vi "Periodic Tasks.vi"(8 "error in":errorcluster) -> ()   [LabVIEW 2013]
doc: "This VI runs in parallel to other tasks. It can contain as many user-defined periodic loops as you need. These can carry out PID or other sorts of timed response."
uses:
  <vilib>/Rock Robotics/SystemInterfaces/Utilities/FPGA_UtilitiesLED Source.ctl
  <vilib>/Rock Robotics/SystemInterfaces/Utilities/FPGA_UtilitiesLED State.ctl
  <vilib>/Rock Robotics/WPI/Relay/WPI_RelayValue.ctl
  <vilib>/Rock Robotics/WPI/Compressor/WPI_CompressorGetSetRefNum.vi
  Robot Global Data.vi
  <vilib>/Rock Robotics/WPI/RobotDrive/WPI_RobotDriveGetSetRefNum.vi
  <vilib>/Rock Robotics/WPI/Joystick/WPI_JoystickGetSetRefNum.vi
panel:
  out "Timings":cluster{"Call Name":string, "Delta (ms)":u32}[](array[cluster])
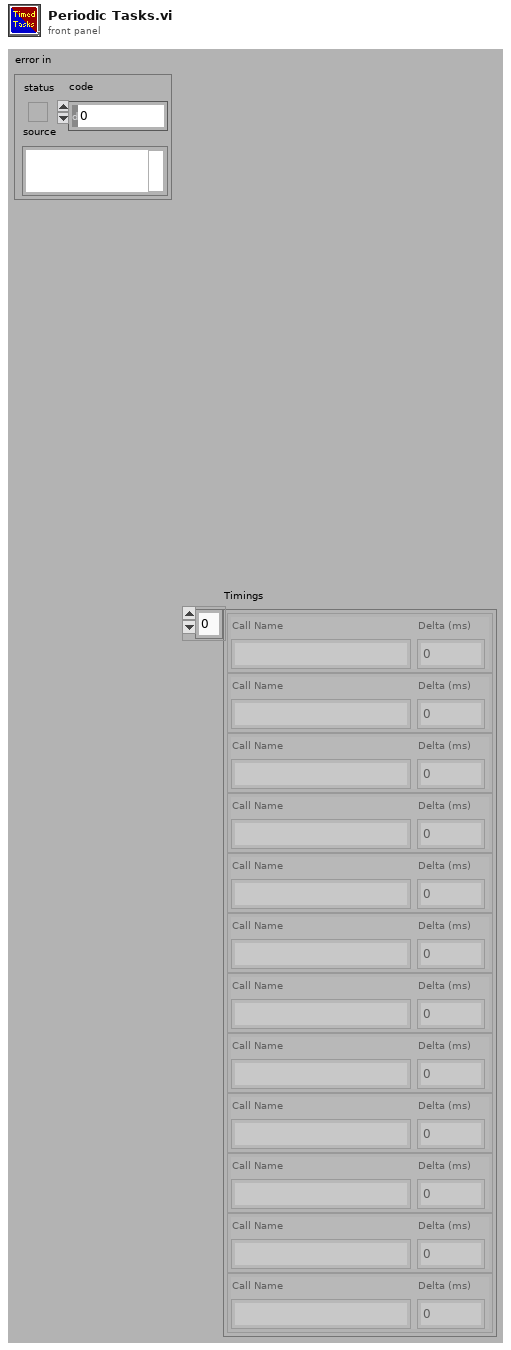
[diagram p1: front panel]
types:
  T1 = typedef "WPI_JoystickDevRef.ctl" = cluster{"Device":T2}
  T2 = typedef "WPI_JoystickDeviceEnum.ctl" = enum16{"USB 1", "USB 2", "USB 3", "USB 4", "Kinect 1", "Kinect 2"}
  T3 = typedef "WPI_RobotDriveDevRef.ctl" = cluster{"DevStatus":errorcluster, "Motors[]":T4[], "Square Inputs":bool, "Max Output":dbl, "Isochronous":bool}
  T4 = typedef "WPI_MotorControlDeviceRef.ctl" = cluster{"DeviceStatus":errorcluster, "Type":enum16{"PWM", "CAN"}, "PWM":cluster{"Digital Module":T5, "PWM Channel":T6, "DeadBand":T7}, "CAN":cluster{"Device Number":u8, "Control Mode":T8, "Semaphore":T9, "Max Vout":dbl}, "Invert":bool, "TransformRef":T10, "InvTransformRef":T10}
  T5 = typedef "FPGA_TypedefDigitalModule.ctl" = enum16{"Digital Module 1", "Digital Module 2"}
  T6 = typedef "FPGA_DIOPWMChannel.ctl" = enum8{"PWM 1", "PWM 2", "PWM 3", "PWM 4", "PWM 5", "PWM 6", "PWM 7", "PWM 8", "PWM 9", "PWM 10", "Invalid"}
  T7 = typedef "WPI_PWMDeadband.ctl" = cluster{"Name":string, "maxPositivePwm":i32, "minPositivePwm":i32, "centerPwm":i32, "maxNegativePwm":i32, "minNegativePwm":i32, "angularRange":u16}
  T8 = typedef "WPI_CANJaguar_ControlMode.ctl" = enum8{"Percent VBus", "Current", "Speed", "Position", "Voltage"}
  T9 = typedef "Semaphore RefNum" = refnum<k1>
  T10 = typedef "WPI_PWMTransform_ConPane.ctl" = refnum<vi>
  T11 = cluster{"JoystickDevRef":T1, "RobotDriveDevRef":T3}
  T12 = typedef "WPI_RelayValue.ctl" = enum16{"Off", "On", "Forward", "Reverse"}
  T13 = typedef "WPI_DriverStationAllianceInfo.ctl" = enum16{"Red", "Blue", "Invalid"}
  T14 = typedef "WPI_RelayDevRef.ctl" = cluster{"DevStatus":errorcluster, "Relay Channel":T15, "Digital Module":T5, "Relay Direction":T16}
  T15 = typedef "FPGA_DIORelayChannel.ctl" = enum8{"Relay 1", "Relay 2", "Relay 3", "Relay 4", "Relay 5", "Relay 6", "Relay 7", "Relay 8", "Invalid"}
  T16 = typedef "WPI_RelayDirection.ctl" = enum16{"Both directions", "Forward only", "Reverse only"}
  T17 = typedef "WPI_CompressorDevRef.ctl" = cluster{"DevStatus":errorcluster, "DigitalInputDevRef":T18, "RelayDevRef":T14}
  T18 = typedef "WPI_DigitalInputDevRef.ctl" = cluster{"DevStatus":errorcluster, "DIO Channel":T19, "Digital Module":T5}
  T19 = typedef "FPGA_DIOChannel.ctl" = enum8{"DIO 1", "DIO 2", "DIO 3", "DIO 4", "DIO 5", "DIO 6", "DIO 7", "DIO 8", "DIO 9", "DIO 10", "DIO 11", "DIO 12", "DIO 13", "DIO 14", "Invalid"}
  T20 = typedef "WPI_JoystickButtonState.ctl" = cluster{"Button 1":bool, "Button 2":bool, "Button 3":bool, "Button 4":bool, "Button 5":bool, "Button 6":bool, "Button 7":bool, "Button 8":bool, "Button 9":bool, "Button 10":bool, "Button 11":bool, "Button 12":bool}
  T21 = cluster{"axis 1 (x)":dbl, "axis 2 (y)":dbl, "axis 3 (throttle)":dbl, "axis 4":dbl, "axis 5":dbl, "axis 6":dbl}
  T22 = typedef "FPGA_UtilitiesLED State.ctl" = enum16{"Off", "On", "Toggle"}
  T23 = typedef "FPGA_UtilitiesLED Source.ctl" = enum16{"User LED", "FPGA LED"}
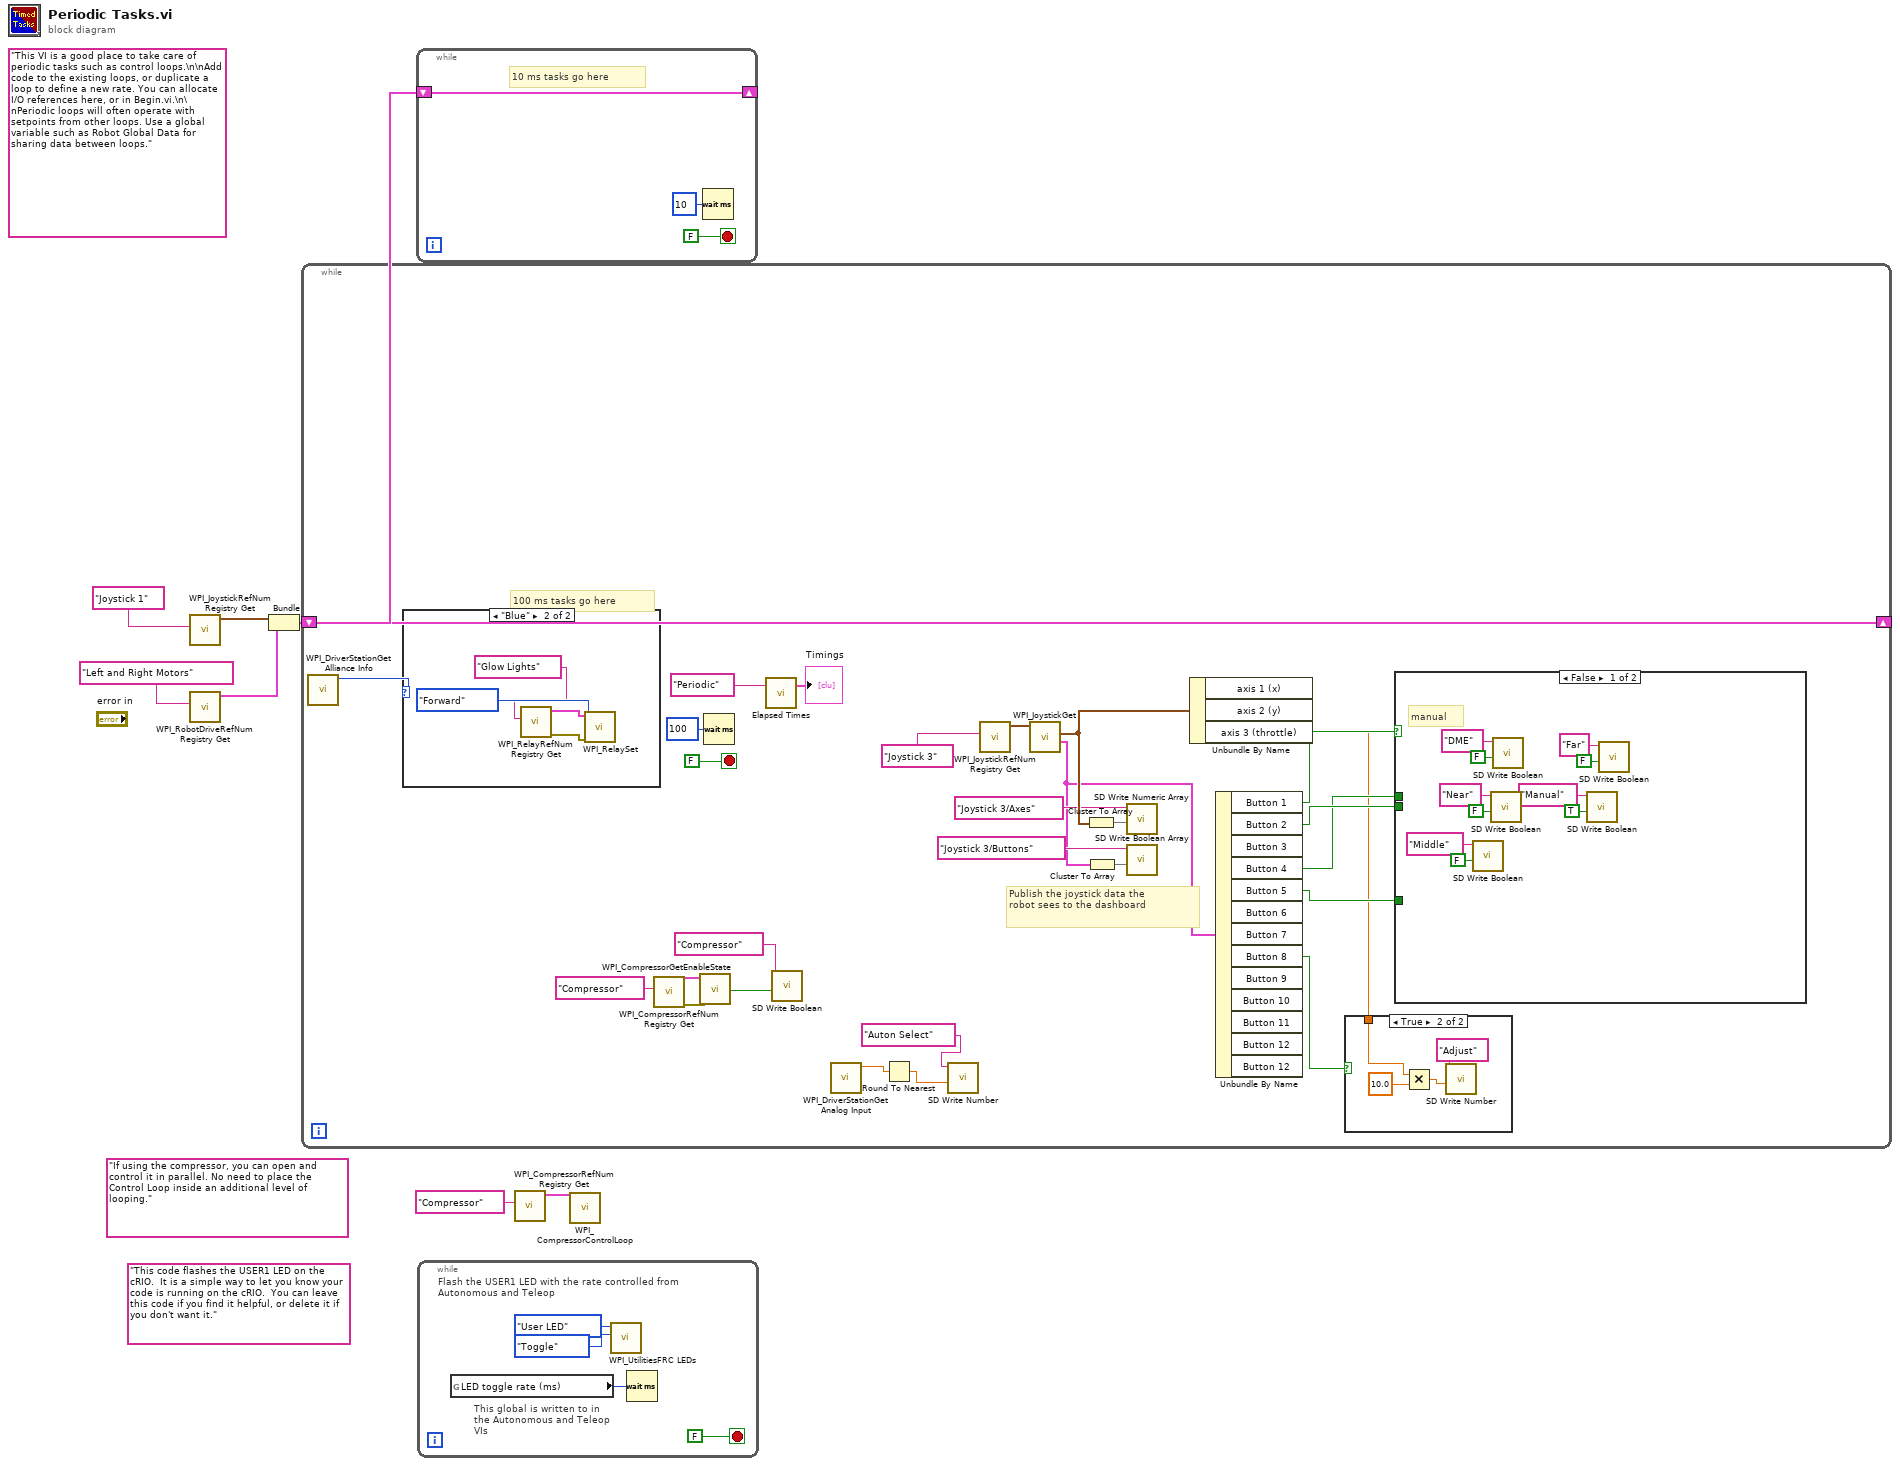
[diagram p0: block diagram]
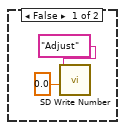
[diagram p2: hidden frame]
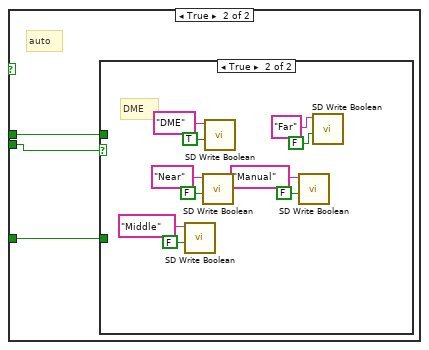
[diagram p3: hidden frame]
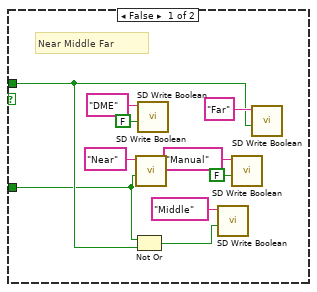
[diagram p4: hidden frame]
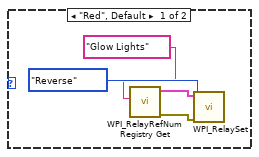
[diagram p5: hidden frame]
diagram:
  (unwired) "If using the compressor, you can open and control it in parallel. No need to place the Control Loop inside an additional level of looping."
  (unwired) "This code flashes the USER1 LED on the cRIO.  It is a simple way to let you know your code is running on the cRIO.  You can leave this code if you find it helpful, or delete it if you don't want it."
  (unwired) "This VI is a good place to take care of periodic tasks such as control loops.\n\nAdd code to the existing loops, or duplicate a loop to define a new rate. You can allocate I/O references here, or in Begin.vi.\n\nPeriodic loops will often operate with setpoints from other loops. Use a global variable such as Robot Global Data for sharing data between loops."
  n1 = call <vilib>:"WPI_JoystickRefNum Registry Get.vi"("refnum name"="Joystick 1") -> ("JoystickDevRef"=w5:T1)  [unwired: 1 in, 9 out]
  n2 = call <vilib>:"WPI_RobotDriveRefNum Registry Get.vi"("refnum name"="Left and Right Motors") -> ("RobotDriveDevRef"=w4:T3)  [unwired: 1 in, 9 out]
  n3 = Bundle("JoystickDevRef"=w5, "RobotDriveDevRef"=w4) -> (w3:T11)  [unwired: 1 out]
  n4 = while {
    shift-right: [w33] -> _
    shift-left: w3 -> [w33]
    stop <- FALSE stop-if-true
    # "Publish the joystick data the\nrobot sees to the dashboard"
    # "100 ms tasks go here"
    n5 = call <vilib>:"WPI_DriverStationGet Alliance Info.vi"() -> ("Alliance"=w32:T13)  [unwired: 10 in, 1 out]
    n6 = case shown="\"Blue\"" w32 {
      frame "Red", Default {
        n7 = call <vilib>:"WPI_RelayRefNum Registry Get.vi"("refnum name"="Glow Lights") -> ("error out"=w77:errorcluster, "RelayDevRef"=w76:T14)  [unwired: 9 in]
        n8 = call <vilib>:"WPI_RelaySet.vi"("error in (no error)"=w77, "RelayValue"=WPI_RelayValue."Reverse", "RelayDevRef"=w76) -> ()  [unwired: 7 in, 2 out]
      }
      frame "Blue" {
        n9 = call <vilib>:"WPI_RelayRefNum Registry Get.vi"("refnum name"="Glow Lights") -> ("error out"=w81:errorcluster, "RelayDevRef"=w80:T14)  [unwired: 9 in]
        n10 = call <vilib>:"WPI_RelaySet.vi"("error in (no error)"=w81, "RelayValue"=WPI_RelayValue."Forward", "RelayDevRef"=w80) -> ()  [unwired: 7 in, 2 out]
      }
    }
    n11 = call <vilib>:"WPI_CompressorRefNum Registry Get.vi"("refnum name"="Compressor") -> ("error out"=w12:errorcluster, "CompressorDevRef"=w11:T17)  [unwired: 9 in]
    n12 = call <vilib>:"WPI_CompressorGetEnableState.vi"("error in (no error)"=w12, "CompressorDevRef"=w11) -> ("Compressor Running"=w9:bool)  [unwired: 6 in, 3 out]
    n13 = Wait (ms)(milliseconds to wait=u32 100) -> ()  [unwired: 1 out]
    n14 = call "Elapsed Times.vi"("Call Name"="Periodic") -> ("Timings"=→"Timings":cluster{"Call Name":string, "Delta (ms)":u32}[])  [unwired: 2 in]
    n15 = call <vilib>:"SD Write Boolean.vi"("Boolean"=w9, "Name"="Compressor") -> ()  [unwired: 8 in, 2 out]
    n16 = call <vilib>:"WPI_DriverStationGet Analog Input.vi"() -> ("Analog 1 (V)"=w16:dbl)  [unwired: 8 in, 3 out]
    n17 = Round To Nearest(number=w16) -> (nearest integer value=w15:dbl)
    n18 = call <vilib>:"SD Write Number.vi"("Numeric"=w15, "Name"="Auton Select") -> ()  [unwired: 8 in, 2 out]
    n19 = call <vilib>:"WPI_JoystickRefNum Registry Get.vi"("refnum name"="Joystick 3") -> ("JoystickDevRef"=w28:T1)  [unwired: 1 in, 9 out]
    n20 = call <vilib>:"WPI_JoystickGet.vi"("JoystickDevRef"=w28) -> ("Buttons"=w22:T20, "Axes"=w25:T21)  [unwired: 1 in, 4 out]
    n21 = Cluster To Array(cluster=w25) -> (array=w24:dbl[])
    n22 = Cluster To Array(cluster=w22) -> (array=w27:bool[])
    n23 = call <vilib>:"SD Write Numeric Array.vi"("Numeric Array"=w24, "Name"="Joystick 3/Axes") -> ()  [unwired: 8 in, 2 out]
    n24 = call <vilib>:"SD Write Boolean Array.vi"("Boolean Array"=w27, "Name"="Joystick 3/Buttons") -> ()  [unwired: 8 in, 2 out]
    n25 = Unbundle By Name(w25) -> ("axis 3 (throttle)"=w13:dbl)  [unwired: 2 out]
    n26 = Unbundle By Name(w22) -> ("Button 1"=w21:bool, "Button 2"=w20:bool, "Button 4"=w18:bool, "Button 5"=w19:bool, "Button 8"=w17:bool)  [unwired: 8 out]
    n27 = case shown="True" w17 {
      tunnel: w13 -> [_ w38]
      frame False {
        n28 = call <vilib>:"SD Write Number.vi"("Numeric"=0.0, "Name"="Adjust") -> ()  [unwired: 8 in, 2 out]
      }
      frame True {
        n29 = Multiply(x=w38, y=10.0) -> (x*y=w41:dbl)
        n30 = call <vilib>:"SD Write Number.vi"("Numeric"=w41, "Name"="Adjust") -> ()  [unwired: 8 in, 2 out]
      }
    }
    n31 = case shown="False" w21 {
      tunnel: w20 -> [_ w54]
      tunnel: w19 -> [_ w53]
      tunnel: w18 -> [_ w52]
      frame False {
        # "manual"
        n32 = call <vilib>:"SD Write Boolean.vi"("Boolean"=FALSE, "Name"="Middle") -> ()  [unwired: 8 in, 2 out]
        n33 = call <vilib>:"SD Write Boolean.vi"("Boolean"=FALSE, "Name"="Near") -> ()  [unwired: 8 in, 2 out]
        n34 = call <vilib>:"SD Write Boolean.vi"("Boolean"=FALSE, "Name"="DME") -> ()  [unwired: 8 in, 2 out]
        n35 = call <vilib>:"SD Write Boolean.vi"("Boolean"=TRUE, "Name"="Manual") -> ()  [unwired: 8 in, 2 out]
        n36 = call <vilib>:"SD Write Boolean.vi"("Boolean"=FALSE, "Name"="Far") -> ()  [unwired: 8 in, 2 out]
      }
      frame True {
        # "auto"
        n37 = case shown="True" w54 {
          tunnel: w53 -> [w56 _]
          tunnel: w52 -> [w57 _]
          frame False {
            # "Near Middle Far"
            n38 = Not Or(1:w57, 2:w56) -> (0:w58:bool)
            n39 = call <vilib>:"SD Write Boolean.vi"("Boolean"=w56, "Name"="Near") -> ()  [unwired: 8 in, 2 out]
            n40 = call <vilib>:"SD Write Boolean.vi"("Boolean"=FALSE, "Name"="DME") -> ()  [unwired: 8 in, 2 out]
            n41 = call <vilib>:"SD Write Boolean.vi"("Boolean"=w58, "Name"="Middle") -> ()  [unwired: 8 in, 2 out]
            n42 = call <vilib>:"SD Write Boolean.vi"("Boolean"=FALSE, "Name"="Manual") -> ()  [unwired: 8 in, 2 out]
            n43 = call <vilib>:"SD Write Boolean.vi"("Boolean"=w57, "Name"="Far") -> ()  [unwired: 8 in, 2 out]
          }
          frame True {
            # "DME"
            n44 = call <vilib>:"SD Write Boolean.vi"("Boolean"=FALSE, "Name"="Middle") -> ()  [unwired: 8 in, 2 out]
            n45 = call <vilib>:"SD Write Boolean.vi"("Boolean"=FALSE, "Name"="Near") -> ()  [unwired: 8 in, 2 out]
            n46 = call <vilib>:"SD Write Boolean.vi"("Boolean"=TRUE, "Name"="DME") -> ()  [unwired: 8 in, 2 out]
            n47 = call <vilib>:"SD Write Boolean.vi"("Boolean"=FALSE, "Name"="Manual") -> ()  [unwired: 8 in, 2 out]
            n48 = call <vilib>:"SD Write Boolean.vi"("Boolean"=FALSE, "Name"="Far") -> ()  [unwired: 8 in, 2 out]
          }
        }
      }
    }
  }
  n49 = while {
    shift-right: [w83] -> _
    shift-left: w3 -> [w83]
    stop <- FALSE stop-if-true
    # "10 ms tasks go here"
    n50 = Wait (ms)(milliseconds to wait=u32 10) -> ()  [unwired: 1 out]
  }
  n51 = while {
    stop <- FALSE stop-if-true
    # "This global is written to in the Autonomous and Teleop VIs"
    # "Flash the USER1 LED with the rate controlled from Autonomous and Teleop"
    n52 = global read "Robot Global Data.vi" "LED toggle rate (ms)"() -> (w86:u32)
    n53 = call <vilib>:"WPI_UtilitiesFRC LEDs.vi"("State"=FPGA_UtilitiesLED_State."Toggle", "LED Type"=FPGA_UtilitiesLED_Source."User LED") -> ()  [unwired: 1 in, 9 out]
    n54 = Wait (ms)(milliseconds to wait=w86) -> ()  [unwired: 1 out]
  }
  n55 = call <vilib>:"WPI_CompressorRefNum Registry Get.vi"("refnum name"="Compressor") -> ("CompressorDevRef"=w1:T17)  [unwired: 9 in, 1 out]
  n56 = call <vilib>:"WPI_CompressorControlLoop.vi"("CompressorDevRef"=w1) -> ()  [unwired: 11 in]
